vi "uNTILTED 3.vi"() -> ()   [LabVIEW 2019]
uses:
  Viejos/Alfredo LABVIEW/Set-up verificador ASICs/Lib Agilent 81160A/Agilent 81150/Agilent 81150.lvlib
panel:
  in  "stop 2":bool
  in  "stop":bool
  out "error out 2":errorcluster
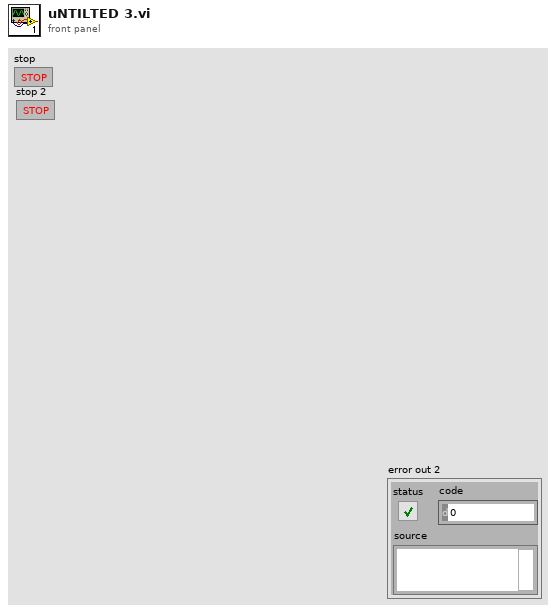
[diagram p1: front panel]
types:
  T1 = enum16{"INIT GEN", "RECORRER TENSIONES", "APAGAR FUENTE Y GEN"}
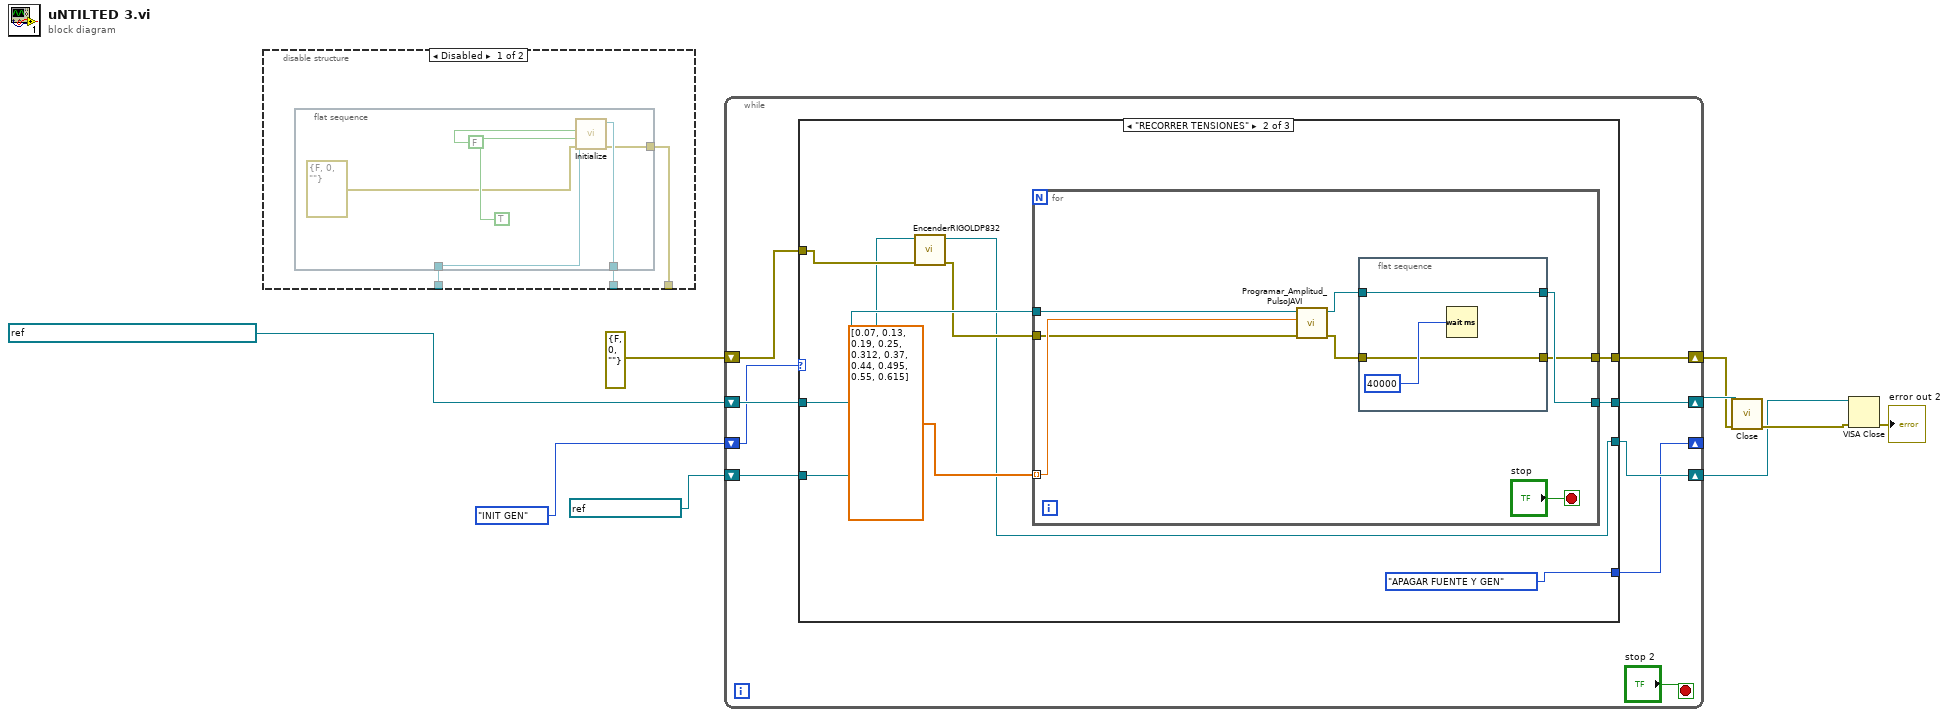
[diagram p0: block diagram]
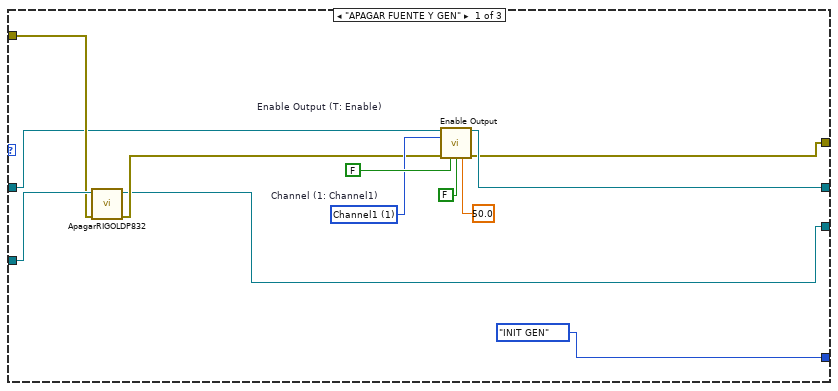
[diagram p3: hidden frame]
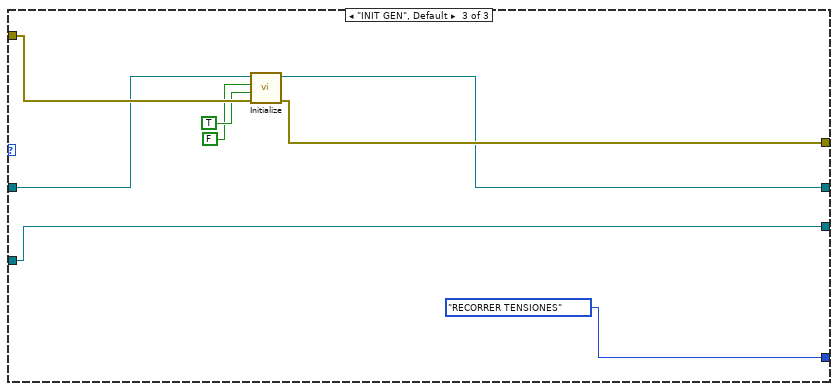
[diagram p4: hidden frame]
diagram:
  n1 = disable-structure shown="Disabled" {
    disable-tunnel: _ -> [w12 _]
    disable-tunnel: [w11 _] -> _
    disable-tunnel: [w10 _] -> _
    frame Disabled {
      n2 = flat-sequence {
        tunnel: w12 -> [w16]
        tunnel: [w15] -> w11
        tunnel: [w14] -> w10
        frame #0 {
          n3 = call "Initialize.vi"("error in (no error)"=errorcluster {"status"=FALSE, "code"=0, "source"=""}, "Reset (True)"=TRUE, "ID Query (True)"=FALSE, "VISA resource name"=w16) -> ("error out"=w14:errorcluster, "VISA resource name out"=w15:refnum<visa-resource-name>)  [unwired: 6 in]
        }
      }
    }
    frame Enabled {
    }
  }
  n4 = while {
    shift-right: [w25] -> w9
    shift-left: refnum<visa-resource-name> "USB0::0x0957::0x4108::MY51400682::INSTR" ("VISA Refnum in") -> [w27]
    shift-right: [w24] -> w8
    shift-left: errorcluster {"status"=FALSE, "code"=0, "source"=""} ("error out") -> [w26]
    shift-right: [w22] -> w5
    shift-left: refnum<visa-resource-name> "FA_Rigol_DP832" ("VISA IN") -> [w23]
    shift-right: [w19] -> _
    shift-left: T1."INIT GEN" ("Enum") -> [w20]
    stop <- "stop 2" stop-if-true
    n5 = case shown="\"RECORRER TENSIONES\"" w20 {
      tunnel: w27 -> [w32 w48 w62]
      tunnel: w26 -> [w38 w44 w67]
      tunnel: [w31 w47 w61] -> w25
      tunnel: [w29 w46 w66] -> w24
      tunnel: w23 -> [w39 w43 w60]
      tunnel: [w30 w41 w60] -> w22
      tunnel: [T1."INIT GEN" ("Enum") T1."APAGAR FUENTE Y GEN" ("Enum") T1."RECORRER TENSIONES" ("Enum")] -> w19
      frame "APAGAR FUENTE Y GEN" {
        w36 = u16 1 items=["Channel1"=1, "Channel2"=2]  # Channel (1: Channel1)
        w37 = FALSE  # Enable Output (T: Enable)
        n6 = call "ApagarRIGOLDP832.vi"("error in (no error)"=w38, "VISA resource name"=w39) -> ("error out"=w33:errorcluster, "VISA resource name out"=w30:refnum<visa-resource-name>)  [unwired: 8 in]
        n7 = call "Enable Output.vi"("VISA resource name"=w32, "Channel (1: Channel1)"=w36, "error in (no error)"=w33, "Enable Output (T: Enable)"=w37, "Enable Output Complement (T: Enable)"=FALSE, "Load (50 Ohm)"=50.0) -> ("VISA resource name out"=w31:refnum<visa-resource-name>, "error out"=w29:errorcluster)  [unwired: 8 in]
      }
      frame "RECORRER TENSIONES" {
        n8 = call "EncenderRIGOLDP832.vi"("error in (no error)"=w44, "VISA IN"=w43) -> ("error out"=w42:errorcluster, "VISA resource name out"=w41:refnum<visa-resource-name>)  [unwired: 8 in]
        n9 = for {
          tunnel: dbl[] [0.07, 0.13, 0.19, 0.25, 0.312, 0.37, 0.44, 0.495, 0.55, 0.615] -> [w56] mode=indexing
          tunnel: w48 -> [w55]
          tunnel: [w52] -> w47
          tunnel: [w51] -> w46
          tunnel: w42 -> [w50]
          stop <- "stop" stop-if-true
          n10 = call "Programar_Amplitud_PulsoJAVI.vi"("error in (no error)"=w50, "Numeric"=w56, "VISA Refnum in"=w55) -> ("Error OUT"=w53:errorcluster, "VISA resource name out"=w54:refnum<visa-resource-name>)  [unwired: 7 in]
          n11 = flat-sequence {
            tunnel: [w58] -> w52
            tunnel: w54 -> [w58]
            tunnel: [w57] -> w51
            tunnel: w53 -> [w57]
            frame #0 {
              n12 = Wait (ms)(milliseconds to wait=u32 40000) -> ()  [unwired: 1 out]
            }
          }
        }
      }
      frame "INIT GEN", Default {
        n13 = call "Initialize.vi"("error in (no error)"=w67, "Reset (True)"=TRUE, "ID Query (True)"=FALSE, "VISA resource name"=w62) -> ("error out"=w66:errorcluster, "VISA resource name out"=w61:refnum<visa-resource-name>)  [unwired: 6 in]
      }
    }
  }
  n14 = call "Close.vi"("error in (no error)"=w8, "VISA resource name"=w9) -> ("error out"=w7:errorcluster)  [unwired: 9 in]
  n15 = VISA Close(VISA resource name=w5, error in (no error)=w7) -> (error out=→"error out 2":errorcluster)
